vi "connect.vi"(6 "timeout ms (10000)":i32=10000, 8 "error in":errorcluster, 11 "Queue client in":refnum<class "Queue client.lvclass">) -> (0 "error out":errorcluster, 1 "valid?":bool, 2 "new connection":refnum<class "connection maintainer.lvclass">, 3 "Queue client out":refnum<class "Queue client.lvclass">)   [LabVIEW 2015, in "Queue client.lvclass"]
uses:
  Queue client.lvclass
  connection/connection maintainer.lvclass
  client/connection client.lvclass/connection client.ctl
  Queue connection/Queue connection.lvclass
  client/connection client.lvclass
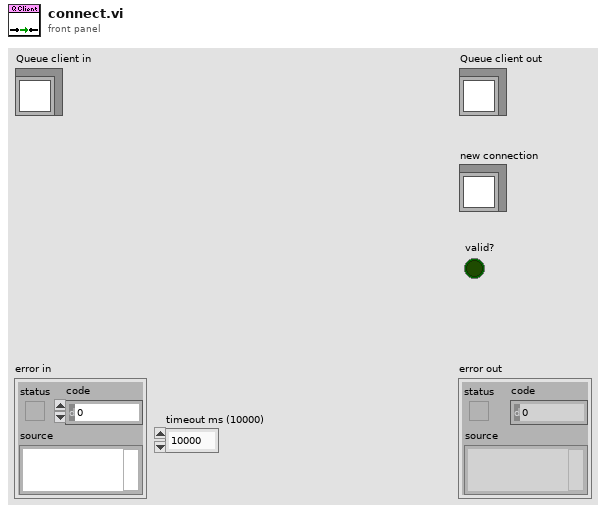
[diagram p1: front panel]
types:
  T1 = typedef "Queue connection.lvclass/queue pair.ctl" = cluster{"to pair":refnum<queue>, "from pair":refnum<queue>}
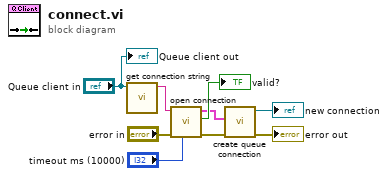
[diagram p0: block diagram]
diagram:
  n1 = call "get connection string.vi"("connection client in"="Queue client in") -> ("connection string"=w1:string)  [unwired: 10 in]
  n2 = call "open connection.vi"("timeout ms (10000)"="timeout ms (10000)", "error in"="error in", "address"=w1) -> ("error out"=w5:errorcluster, "valid?"=→"valid?":bool, "output cluster"=w6:T1)  [unwired: 6 in]
  n3 = call "create queue connection.vi"("error in"=w5, "queues"=w6) -> ("error out"=→"error out":errorcluster, "TCP connection out"=→"new connection":refnum<class "Queue connection.lvclass">)  [unwired: 8 in]
  "Queue client out" <- "Queue client in"
